vi "SMTP Email TCP Read xTP Reply.vi"(8 "error in (no error)":errorcluster, 11 "buffered tcp connection":refnum<k5>) -> (0 "error out":errorcluster, 1 "reply code":i32, 2 "reply string":string, 3 "buffered tcp connection out":refnum<k5>)   [LabVIEW 2012, in "NewNI_SMTPEmail.lvlib"]
doc: "Reads lines from a connection created with TCP Buffered Open.\nThe data is assumed to be in the response format used by FTP, SMTP, etc.\nWhen a line that begins with three digits followed by a space is encountered, all the lines (including this last one) are returned in \"reply string\". The number is returned in \"reply code\"."
uses:
  NewNI_SMTPEmail.lvlib
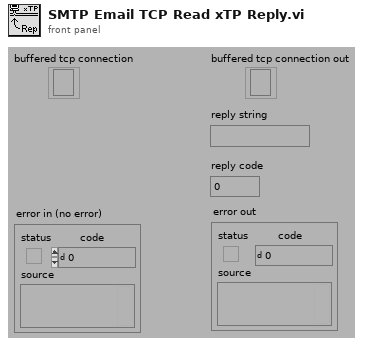
[diagram p1: front panel]
types:
  T1 = enum16{"Standard", "Buffered", "CRLF", "Immediate"}
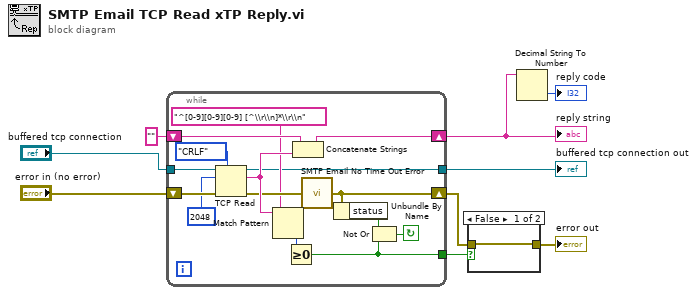
[diagram p0: block diagram]
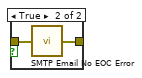
[diagram p2: hidden frame]
diagram:
  n1 = while {
    tunnel: [w12] -> w3
    tunnel: [w13] -> w5
    tunnel: "buffered tcp connection" -> [w19]
    shift-left: "error in (no error)" -> [w20]
    shift-right: [w22] -> w1
    shift-left: "" ("after substring") -> [w17]
    shift-right: [w15] -> w7
    stop <- w23 continue-if-true
    n2 = TCP Read(connection ID=w19, bytes to read=2048, error in (no error)=w20, 7:T1."CRLF" ("mode (standard)")) -> (connection ID out=w13:refnum<k5>, data out=w18:string, error out=w16:errorcluster)  [unwired: 1 out]
    n3 = Match Pattern(string=w18, regular expression="^[0-9][0-9][0-9] [^\\r\\n]*\\r\\n") -> (offset past match=w21:i32)  [unwired: 4 out]
    n4 = Greater Or Equal To 0?(x=w21) -> (x >= 0?=w12:bool)
    n5 = Concatenate Strings(w17, w18) -> (w15:string)
    n6 = call "SMTP Email No Time Out Error.vi"("error in (no error)"=w16) -> ("error out"=w22:errorcluster)  [unwired: 14 out]
    n7 = Unbundle By Name(w22) -> ("status"=w24:bool)
    n8 = Not Or(1:w12, 2:w24) -> (0:w23:bool)
  }
  "buffered tcp connection out" <- w5
  "reply string" <- w7
  n9 = case shown="False" w3 {
    tunnel: w1 -> [w25 w27]
    tunnel: [w25 w26] -> w2
    frame False {
    }
    frame True {
      n10 = call "SMTP Email No EOC Error.vi"("error in (no error)"=w27) -> ("error out"=w26:errorcluster)  [unwired: 4 out]
    }
  }
  "error out" <- w2
  n11 = Decimal String To Number(string=w7) -> (number=→"reply code":i32)  [unwired: 3 out]
